vi "ReadModelData.vi"(8 "error in (no error)":errorcluster, 10 "meas_timestamp in":timestamp, 11 "NHRDCModel in":refnum<class "NHRDCPowerModel.lvclass">) -> (0 "error out":errorcluster, 2 "Model2ICDAS Array":T1[](array[typedef]), 3 "NHRDCModel out":refnum<class "NHRDCPowerModel.lvclass">)   [LabVIEW 2018, in "AcPwrPlugins.lvlib" / "NHRDCPowerModel.lvclass"]
uses:
  NHRDCPowerModel.lvclass
  TypeDefs/NHRDC_Model2ICDAS.ctl
  NHRDCPowerModel.lvclass/NHRDCPowerModel.ctl
  <vilib>/addons/database/_DB Variant To Data/Database Variant To Data.xnode
  Database/DatabaseBaseClass/DatabaseBaseClass.lvclass
  <vilib>/addons/database/NI_Database_API.lvlib
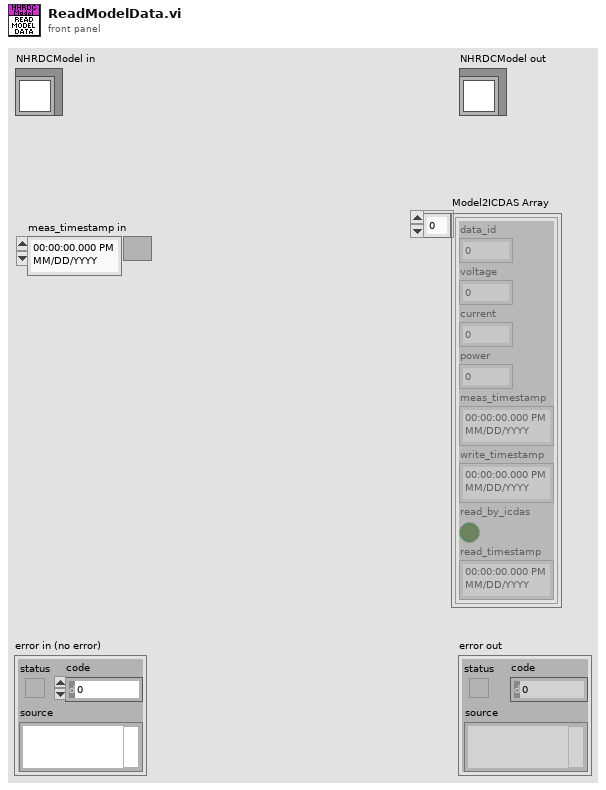
[diagram p1: front panel]
types:
  T1 = typedef "AcPwrPlugins.lvlib/NHRDCPowerModel.lvclass/NHRDC_Model2ICDAS.ctl" = cluster{"data_id":i32, "voltage":dbl, "current":dbl, "power":dbl, "meas_timestamp":timestamp, "write_timestamp":timestamp, "read_by_icdas":bool, "read_timestamp":timestamp}
  T2 = typedef "NI_Database_API.lvlib/Conn ObjectReference.ctl" = refnum<k1>
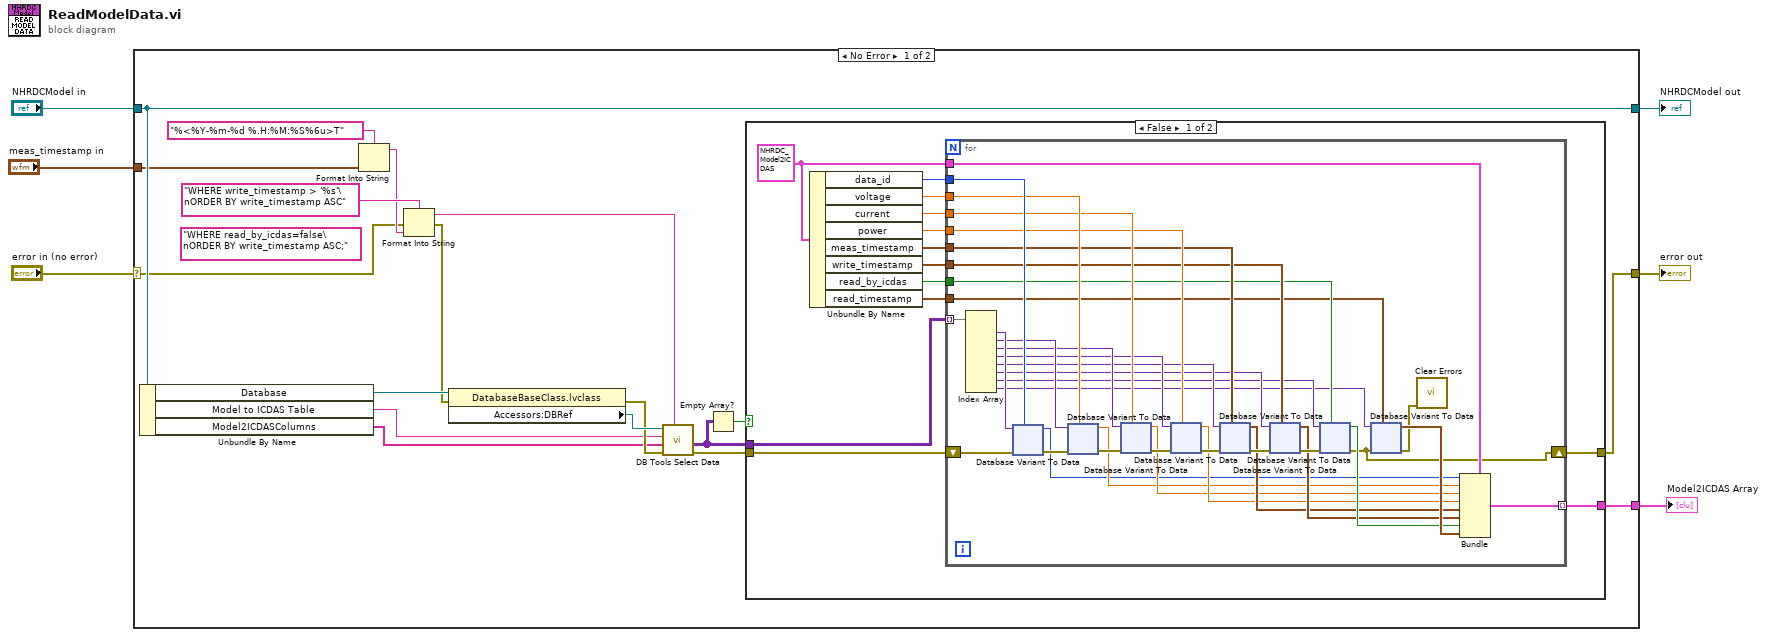
[diagram p0: block diagram]
diagram:
  n1 = case shown="No Error" "error in (no error)" {
    selector: "error in (no error)" -> [w13 w371]
    tunnel: [w7 w371] -> w5
    tunnel: [w24 w370] -> w3
    tunnel: "NHRDCModel in" -> [w24 w370]
    tunnel: "meas_timestamp in" -> [w22 _]
    tunnel: [w8 _] -> w1
    frame No Error {
      (unwired) "WHERE read_by_icdas=false\nORDER BY write_timestamp ASC;" ("condition")
      n2 = Unbundle By Name(w24) -> ("Database"=w19:refnum<class "DatabaseBaseClass.lvclass">, "Model to ICDAS Table"=w15:string, "Model2ICDASColumns"=w14:string[])
      n3 = Format Into String(format string="%<%Y-%m-%d %.H:%M:%S%6u>T", w22) -> (resulting string=w20:string)  [unwired: 2 in, 1 out]
      n4 = Format Into String(format string="WHERE write_timestamp > '%s'\nORDER BY write_timestamp ASC" ("condition"), error in=w13, w20) -> (resulting string=w16:string, error out=w12:errorcluster)  [unwired: 1 in]
      n5 = property class="DatabaseBaseClass.lvclass"(reference=w19, error in=w12) -> (error out=w17:errorcluster, "Accessors:DBRef"=w18:T2)  [unwired: 1 out]
      n6 = call <vilib>:"DB Tools Select Data.vi"("condition"=w16, "error in (no error)"=w17, "columns"=w14, "table"=w15, "connection reference"=w18) -> ("error out"=w11:errorcluster, "data"=w9:variant[][])  [unwired: 1 in, 1 out]
      n7 = Empty Array?(array=w9) -> (empty?=w10:bool)
      n8 = case shown="False" w10 {
        tunnel: w9 -> [w36 _]
        tunnel: w11 -> [w27 w369]
        tunnel: [w25 w369] -> w7
        tunnel: [w26 _] -> w8
        frame False {
          w37 = T1 {"data_id"=0, "voltage"=0.0, "current"=0.0, "power"=0.0, "meas_timestamp"=timestamp(0 s since 1904-01-01), "write_timestamp"=timestamp(0 s since 1904-01-01), "read_by_icdas"=FALSE, "read_timestamp"=timestamp(0 s since 1904-01-01)} ("NHRDC_Model2ICDAS")
          n9 = Unbundle By Name(w37) -> ("data_id"=w35:i32, "voltage"=w34:dbl, "current"=w33:dbl, "power"=w32:dbl, "meas_timestamp"=w31:timestamp, "write_timestamp"=w30:timestamp, "read_by_icdas"=w29:bool, "read_timestamp"=w28:timestamp)
          n10 = for {
            tunnel: w37 -> [w49]
            tunnel: w36 -> [w73] mode=indexing
            tunnel: w35 -> [w71]
            tunnel: w34 -> [w68]
            tunnel: w33 -> [w66]
            tunnel: w32 -> [w64]
            tunnel: w31 -> [w62]
            tunnel: w30 -> [w61]
            tunnel: w29 -> [w58]
            tunnel: w28 -> [w56]
            shift-right: [w39] -> w25
            shift-left: w27 -> [w72]
            tunnel: [w40] -> w26 mode=indexing
            n11 = Index Array(array=w73) -> (element #1=w70:variant, element #2=w67:variant, element #3=w65:variant, element #4=w63:variant, element #5=w60:variant, element #6=w59:variant, element #7=w57:variant, element #8=w55:variant)  [unwired: 8 in]
            n12 = xnode "Database Variant To Data"("database variant"=w70, "error in (no error)"=w72, "type"=w71) -> ("data"=w41:i32, "error out"=w69:errorcluster)
            n13 = xnode "Database Variant To Data"("database variant"=w67, "error in (no error)"=w69, "type"=w68) -> ("data"=w42:dbl, "error out"=w54:errorcluster)
            n14 = xnode "Database Variant To Data"("database variant"=w65, "error in (no error)"=w54, "type"=w66) -> ("data"=w43:dbl, "error out"=w53:errorcluster)
            n15 = xnode "Database Variant To Data"("database variant"=w63, "error in (no error)"=w53, "type"=w64) -> ("data"=w44:dbl, "error out"=w52:errorcluster)
            n16 = xnode "Database Variant To Data"("database variant"=w60, "error in (no error)"=w52, "type"=w62) -> ("data"=w45:timestamp, "error out"=w51:errorcluster)
            n17 = xnode "Database Variant To Data"("database variant"=w59, "error in (no error)"=w51, "type"=w61) -> ("data"=w46:timestamp, "error out"=w50:errorcluster)
            n18 = xnode "Database Variant To Data"("database variant"=w57, "error in (no error)"=w50, "type"=w58) -> ("data"=w47:bool, "error out"=w39:errorcluster)
            n19 = xnode "Database Variant To Data"("database variant"=w55, "error in (no error)"=w39, "type"=w56) -> ("data"=w48:timestamp, "error out"=w38:errorcluster)
            n20 = call <vilib>:"Clear Errors.vi"("error in (no error)"=w38) -> ()  [unwired: 5 in, 2 out]
            n21 = Bundle(cluster=w49, "data_id"=w41, "voltage"=w42, "current"=w43, "power"=w44, "meas_timestamp"=w45, "write_timestamp"=w46, "read_by_icdas"=w47, "read_timestamp"=w48) -> (w40:T1)
          }
        }
        frame True {
        }
      }
    }
    frame Error {
    }
  }
  "error out" <- w5
  "NHRDCModel out" <- w3
  "Model2ICDAS Array" <- w1
